vi "Simulate DMM Multi-Point Reading.vi"() -> ()   [LabVIEW 2013]
panel:
  in  "myDMM_MPReading":dbl[](array[numeric])
  in  "Stop Button":bool
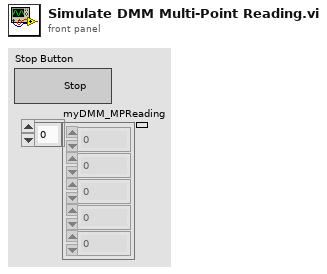
[diagram p1: front panel]
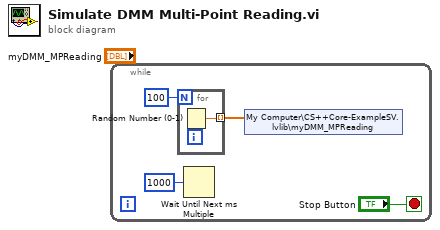
[diagram p0: block diagram]
diagram:
  n1 = while {
    stop <- "Stop Button" stop-if-true
    n2 = for {
      N: 100 -> [_]
      tunnel: [w5] -> w4 mode=indexing
      n3 = Random Number (0-1)() -> (number: 0 to 1=w5:dbl)
    }
    n4 = Wait Until Next ms Multiple(millisecond multiple=u32 1000) -> ()  [unwired: 1 out]
    n5 = shared-variable "My Computer\\CS++Core-ExampleSV.lvlib\\myDMM_MPReading"(w4) -> ()  [unwired: 1 in, 1 out]
  }
